vi "configure.vi"(8 "error in (no error)":errorcluster, 11 "GenericObjective in":refnum<class "GenericObjective.lvclass">) -> (0 "error out":errorcluster, 3 "GenericObjective out":refnum<class "GenericObjective.lvclass">)   [LabVIEW 2010, in "GenericObjective.lvclass"]
doc: "The dynamic dispatch version of this VI loads and displays the configuration file associated with the plug-in object. The user modify and save the configuration data."
uses:
  GenericObjective.lvclass
  correction_enum.ctl
  immersion_enum.ctl
  GenericObjective.lvclass/GenericObjective.ctl
  common/classes/GenericComponent/GenericComponent/GenericComponent.lvclass
panel:
  in  "Tab Control":enum32{"Description", "Configuration settings"}(tab)
  out "Configuration":string
  in  "WorkingDistance":dbl[unit]
  in  "SerialNumber":string
  in  "NominalMagnification":i32
  in  "Model":string
  in  "Manufacturer":string
  in  "LensNA":dbl
  in  "Immersion":T1
  in  "Correction":T2
  in  "CalibratedMagnification":dbl
  out "LSID":string
  in  "save":bool
  in  "cancel":bool
  # "Configure GenericObjective"
  # "The GenericObjective component encapsulates a microscope objective and hold various information about the objective."
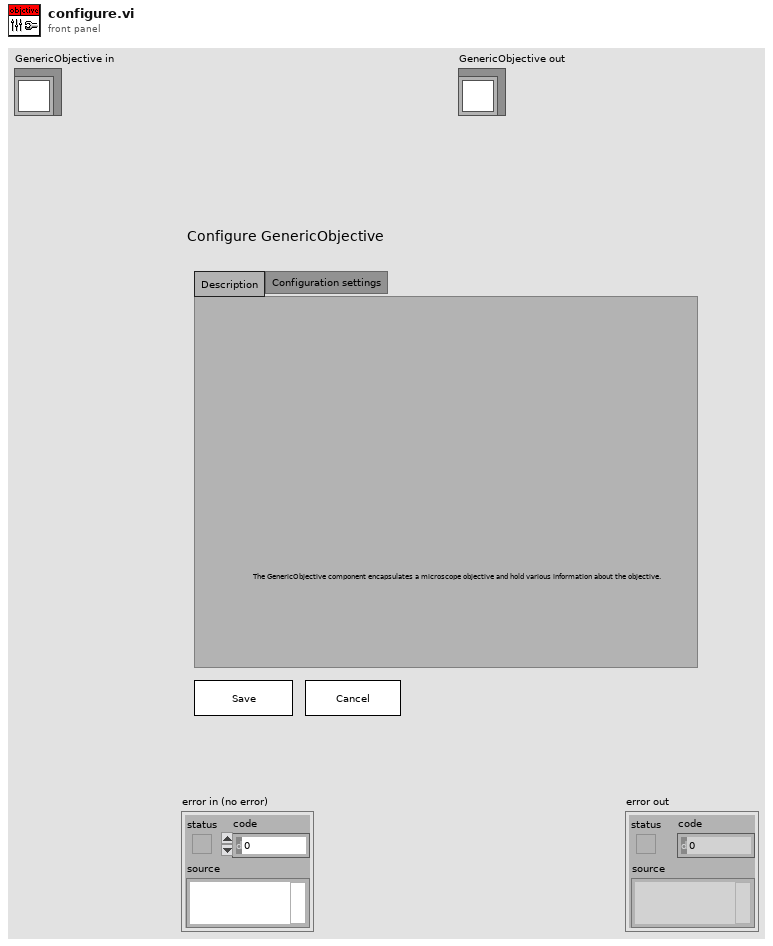
[diagram p1: front panel]
types:
  T1 = typedef "GenericObjective.lvclass/immersion_enum.ctl" = enum16{"Oil", "Water", "WaterDipping", "Air", "Multi", "Glycerol", "Other", "Unknown"}
  T2 = typedef "GenericObjective.lvclass/correction_enum.ctl" = enum16{"UV", "PlanApo", "PlanFluor", "SuperFluor", "VioletCorrected", "Unknown"}
  T3 = typedef "LSID_cluster.ctl" = cluster{"identifier":string, "revision":i32}
  T4 = typedef "GenericObjective.lvclass/config_data_cluster.ctl" = cluster{"LSID":T3, "manufacturer specification":T5, "lens NA":dbl, "nominal magnification":i32, "calibrated magnification":dbl, "working distance":dbl[unit], "correction":T2, "immersion":T1}
  T5 = typedef "manufacturer_specification_cluster.ctl" = cluster{"manufacturer":string, "model":string, "serial number":string, "lot number":string}
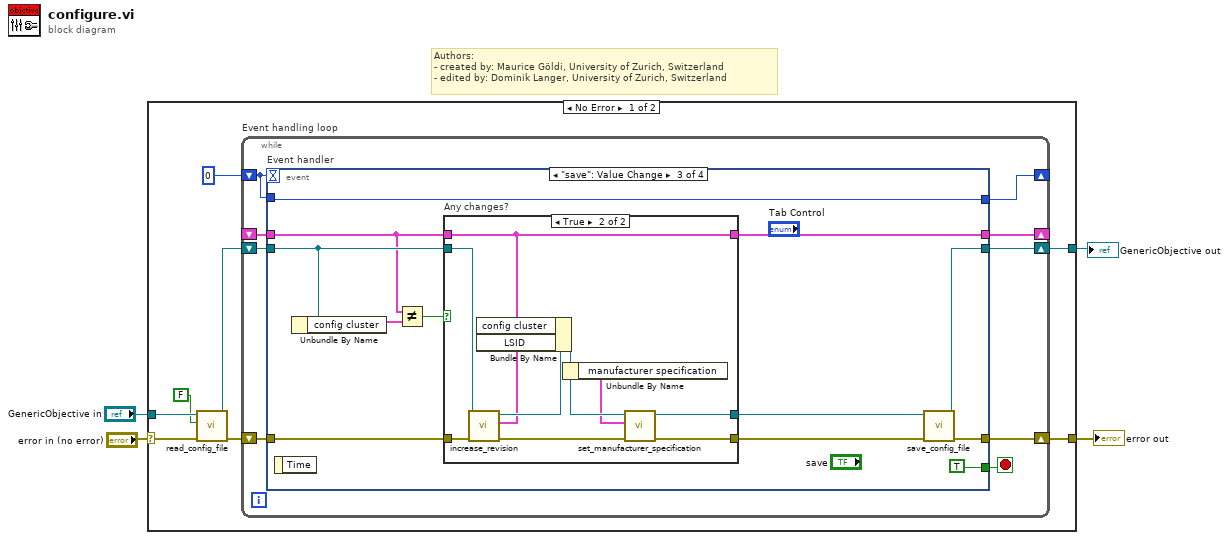
[diagram p0: block diagram]
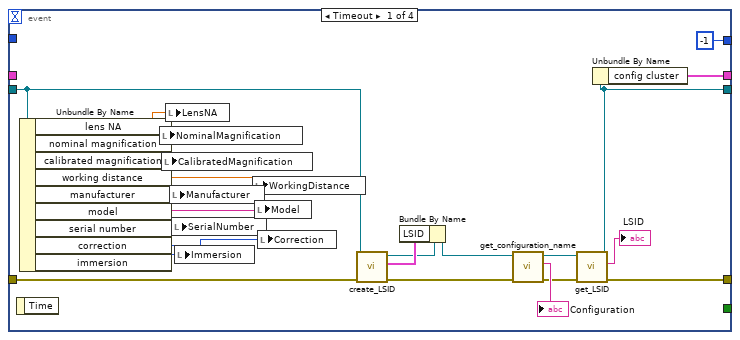
[diagram p2: hidden frame]
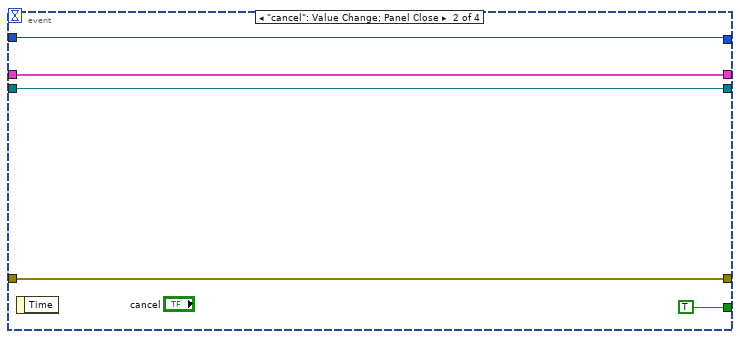
[diagram p3: hidden frame]
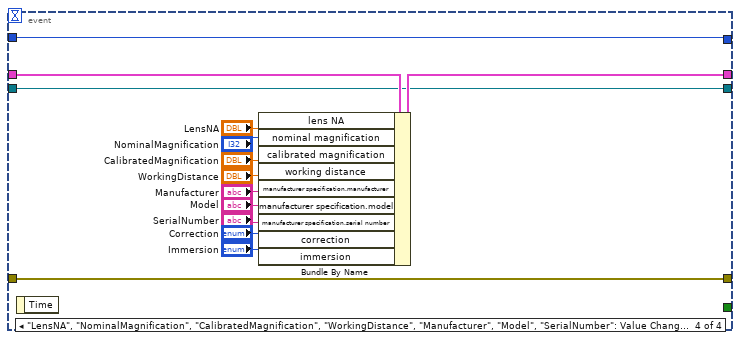
[diagram p5: hidden frame]
diagram:
  # "Authors: \n- created by: Maurice Göldi, University of Zurich, Switzerland\n- edited by: Dominik Langer, University of Zurich, Switzerland"
  n1 = case shown="No Error" "error in (no error)" {
    selector: "error in (no error)" -> [w9 w90]
    tunnel: [w11 w90] -> w3
    tunnel: [w10 w89] -> w1
    tunnel: "GenericObjective in" -> [w7 w89]
    frame No Error {
      n2 = call-dynamic "read_config_file.vi"("error in (no error)"=w9, "force load?"=FALSE, "GenericPlugin in"=w7) -> ("error out"=w5:errorcluster, "GenericPlugin out"=w8:refnum<class "GenericObjective.lvclass">)  [unwired: 7 in]
      n3 = while "Event handling loop" {
        shift-right: [w20] -> _
        shift-left: 0 -> [w21]
        shift-right: [w16] -> w10
        shift-left: w8 -> [w17]
        shift-right: [w18] -> w11
        shift-left: w5 -> [w19]
        shift-right: [w13] -> _
        shift-left: _ -> [w14]
        stop <- w15 stop-if-true
        n4 = event "Event handler" shown="[2] \"save\": Value Change" {
          selector: _ -> [_ _ _ _]
          dyn-events: _ -> [_ _ _ _]
          timeout: w21 -> [_ _ _ _]
          tunnel: w21 -> [_ w46 w61 w88]
          tunnel: [-1 w46 w61 w88] -> w20
          tunnel: [w34 w48 w59 w78] -> w18
          tunnel: w19 -> [w31 w48 w57 w78]
          tunnel: w17 -> [w30 w47 w53 w75]
          tunnel: [w28 w47 w60 w75] -> w16
          tunnel: [_ TRUE TRUE _] -> w15
          tunnel: w14 -> [_ w45 w52 w77]
          tunnel: [w27 w45 w51 w76] -> w13
          event Timeout {
            n5 = event-data() -> ()  [unwired: 1 in, 1 out]
            n6 = Unbundle By Name(w30) -> ("lens NA"=w42:dbl, "nominal magnification"=w32:i32, "calibrated magnification"=w41:dbl, "working distance"=w40:dbl[unit], "manufacturer"=w39:string, "model"=w38:string, "serial number"=w37:string, "correction"=w26:T2, "immersion"=w25:T1)
            n7 = local write "NominalMagnification"(w32) -> ()
            n8 = local write "CalibratedMagnification"(w41) -> ()
            n9 = local write "LensNA"(w42) -> ()
            n10 = local write "Manufacturer"(w39) -> ()
            n11 = local write "SerialNumber"(w37) -> ()
            n12 = local write "Immersion"(w25) -> ()
            n13 = local write "WorkingDistance"(w40) -> ()
            n14 = local write "Model"(w38) -> ()
            n15 = local write "Correction"(w26) -> ()
            n16 = call-dynamic "create_LSID.vi"("error in (no error)"=w31, "GenericPlugin in"=w30) -> ("error out"=w24:errorcluster, "current LSID"=w29:T3, "GenericPlugin out"=w23:refnum<class "GenericObjective.lvclass">)  [unwired: 7 in]
            n17 = Bundle By Name(cluster=w23, "LSID"=w29) -> (w22:refnum<class "GenericObjective.lvclass">)
            n18 = call "get_configuration_name.vi"("error in (no error)"=w24, "GenericPlugin.lvclass in"=w22) -> ("error out"=w35:errorcluster, "configuration name"=→"Configuration":string, "GenericPlugin.lvclass out"=w33:refnum<class "GenericObjective.lvclass">)  [unwired: 7 in]
            n19 = call-dynamic "get_LSID.vi"("error in (no error)"=w35, "GenericPlugin in"=w33) -> ("error out"=w34:errorcluster, "LSID (string)"=→"LSID":string, "GenericPlugin out"=w28:refnum<class "GenericObjective.lvclass">)  [unwired: 6 in, 1 out]
            n20 = Unbundle By Name(w28) -> ("config cluster"=w27:T4)
          }
          event "cancel": Value Change; Panel Close {
            n21 = event-data() -> ()  [unwired: 1 in, 1 out]
          }
          event "save": Value Change {
            n22 = event-data() -> ()  [unwired: 1 in, 1 out]
            n23 = Unbundle By Name(w53) -> ("config cluster"=w55:T4)
            n24 = Not Equal?(x=w52, y=w55) -> (x != y?=w54:bool)
            n25 = case "Any changes?" shown="True" w54 {
              tunnel: w57 -> [w64 w74]
              tunnel: [w64 w68] -> w56
              tunnel: w53 -> [w63 w73]
              tunnel: [w63 w67] -> w50
              tunnel: w52 -> [w62 w70]
              tunnel: [w62 w70] -> w51
              frame False {
              }
              frame True {
                n26 = call-dynamic "increase_revision.vi"("error in (no error)"=w74, "GenericPlugin in"=w73) -> ("error out"=w69:errorcluster, "new LSID"=w71:T3, "GenericPlugin out"=w72:refnum<class "GenericObjective.lvclass">)  [unwired: 7 in]
                n27 = Bundle By Name(cluster=w72, "config cluster"=w70, "LSID"=w71) -> (w66:refnum<class "GenericObjective.lvclass">)
                n28 = Unbundle By Name(w66) -> ("manufacturer specification"=w65:T5)
                n29 = call-dynamic "set_manufacturer_specification.vi"("error in (no error)"=w69, "manufacturer specification"=w65, "GenericPlugin in"=w66) -> ("error out"=w68:errorcluster, "GenericPlugin out"=w67:refnum<class "GenericObjective.lvclass">)  [unwired: 7 in]
              }
            }
            n30 = call-dynamic "save_config_file.vi"("error in (no error)"=w56, "GenericPlugin in"=w50) -> ("error out"=w59:errorcluster, "GenericPlugin out"=w60:refnum<class "GenericObjective.lvclass">)  [unwired: 8 in]
          }
          event "LensNA", "NominalMagnification", "CalibratedMagnification", "WorkingDistance", "Manufacturer", "Model", "SerialNumber": Value Change {
            n31 = event-data() -> ()  [unwired: 1 in, 1 out]
            n32 = Bundle By Name(cluster=w77, "lens NA"="LensNA", "nominal magnification"="NominalMagnification", "calibrated magnification"="CalibratedMagnification", "working distance"="WorkingDistance", "manufacturer specification.manufacturer"="Manufacturer", "manufacturer specification.model"="Model", "manufacturer specification.serial number"="SerialNumber", "correction"="Correction", "immersion"="Immersion") -> (w76:T4)
          }
        }
      }
    }
    frame Error {
    }
  }
  "error out" <- w3
  "GenericObjective out" <- w1
